vi "GT Get Servo Time.vi"(7 "pStepCoef":i32, 8 "error in (no error)":errorcluster caption="错误输入（无错误）", 9 "pDelay":i32, 10 "pServoTime":i32, 11 "cardNum":i16) -> (0 "error out":errorcluster caption="错误输出", 1 "pDelay out":i32, 2 "pServoTime out":i32, 3 "function return":i16, 5 "pStepCoef out":i32)   [LabVIEW 2020, in "gts1.lvlib"]
doc: "GT_API GT_GetServoTime(short cardNum,long *pServoTime,long *pDelay,long *pStepCoef);"
uses:
  gts1.lvlib
  dll/32bit/multi_card/gts.dll
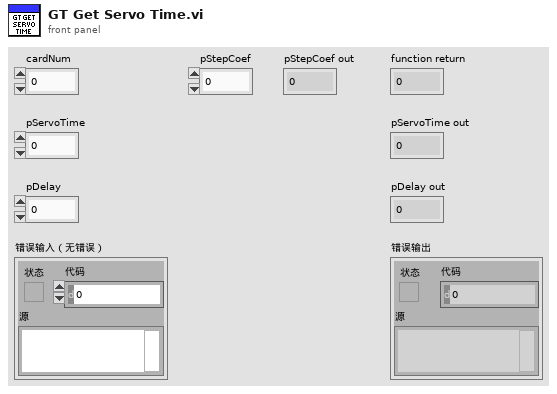
[diagram p1: front panel]
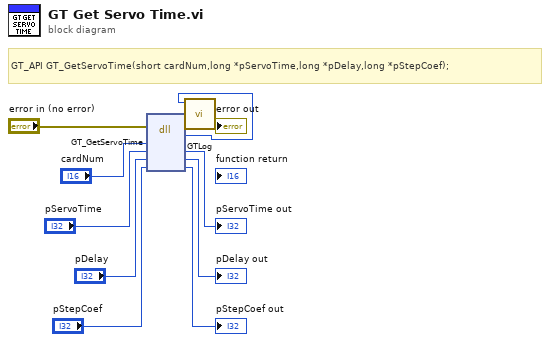
[diagram p0: block diagram]
diagram:
  # "GT_API GT_GetServoTime(short cardNum,long *pServoTime,long *pDelay,long *pStepCoef);"
  n1 = dll-call lib="C:/1228/dll/32bit/multi_card/gts.dll" fn="GT_GetServoTime"(error in="error in (no error)", "cardNum"="cardNum", "pServoTime"="pServoTime", "pDelay"="pDelay", "pStepCoef"="pStepCoef") -> (error out=w3:errorcluster, w1:i16, "pServoTime"=→"pServoTime out":i32, "pDelay"=→"pDelay out":i32, "pStepCoef"=→"pStepCoef out":i32)  [unwired: 3 in, 1 out]
  n2 = call "GTLog.vi"("error in (no error)"=w3, "Numeric"=w1) -> ("error out"=→"error out":errorcluster)  [unwired: 9 in]
